vi "Handle SUBSCRIBED.vi"(0 "reference":refnum<class "WAMP Client.lvclass">, 5 "WAMP Message":T1 {"Message Codes" items=["HELLO"=1, "WELCOME"=2, "ABORT"=3, "GOODBYE"=6, "ERROR"=8, "PUBLISH"=16, "PUBLISHED"=17, "SUBSCRIBE"=32, "SUBSCRIBED"=33, "UNSUBSCRIBE"=34, "UNSUBSCRIBED"=35, "EVENT"=36, "CALL"=48, "RESULT"=59, "REGISTER"=64, "REGISTERED"=65, "UNREGISTER"=66, "UNREGISTERED"=67, "INVOCATION"=68, "YIELD"=70]}, 9 "Subscription Requests In":T3, 11 "error in (no error)":errorcluster) -> (4 "reference out":refnum<class "WAMP Client.lvclass">, 10 "Message Loop Data (out)":T3, 15 "error out":errorcluster)   [LabVIEW 2020, in "wamplv.lvlib" / "WAMP Client.lvclass"]
uses:
  WAMP Client.lvclass
  TypeDef/Message Loop Shift Reg Data.ctl
  TypeDef/REGISTER Request Data.ctl
  TypeDef/Success or error.ctl
  TypeDef/Combined error.ctl
  TypeDef/WAMP Error Payload.ctl
  TypeDef/INVOCATION payload.ctl
  TypeDef/Publish Requests Map.ctl
  TypeDef/PUBLISH Request Data.ctl
  TypeDef/PUBLISH Result.ctl
  TypeDef/Endpoint Data.ctl
  TypeDef/CALL Request Map.ctl
  TypeDef/CALL Request Data.ctl
  TypeDef/RESULT Payload.ctl
  TypeDef/SUBSCRIBE Requests Map.ctl
  TypeDef/SUBSCRIBE Request Data.ctl
  TypeDef/Subscribe Result.ctl
  TypeDef/Event Payload.ctl
  TypeDef/Subscriptions Map.ctl
  TypeDef/Subscription Details.ctl
  TypeDef/Unsubscribe Requests Map.ctl
  TypeDef/UNSUBSCRIBE Request Data.ctl
  TypeDef/UNSUBSCRIBE Result.ctl
  TypeDef/Unregister requests map.ctl
  TypeDef/Unregister request.ctl
  TypeDef/WAMP Received Message.ctl
  TypeDef/WAMP Message Codes.ctl
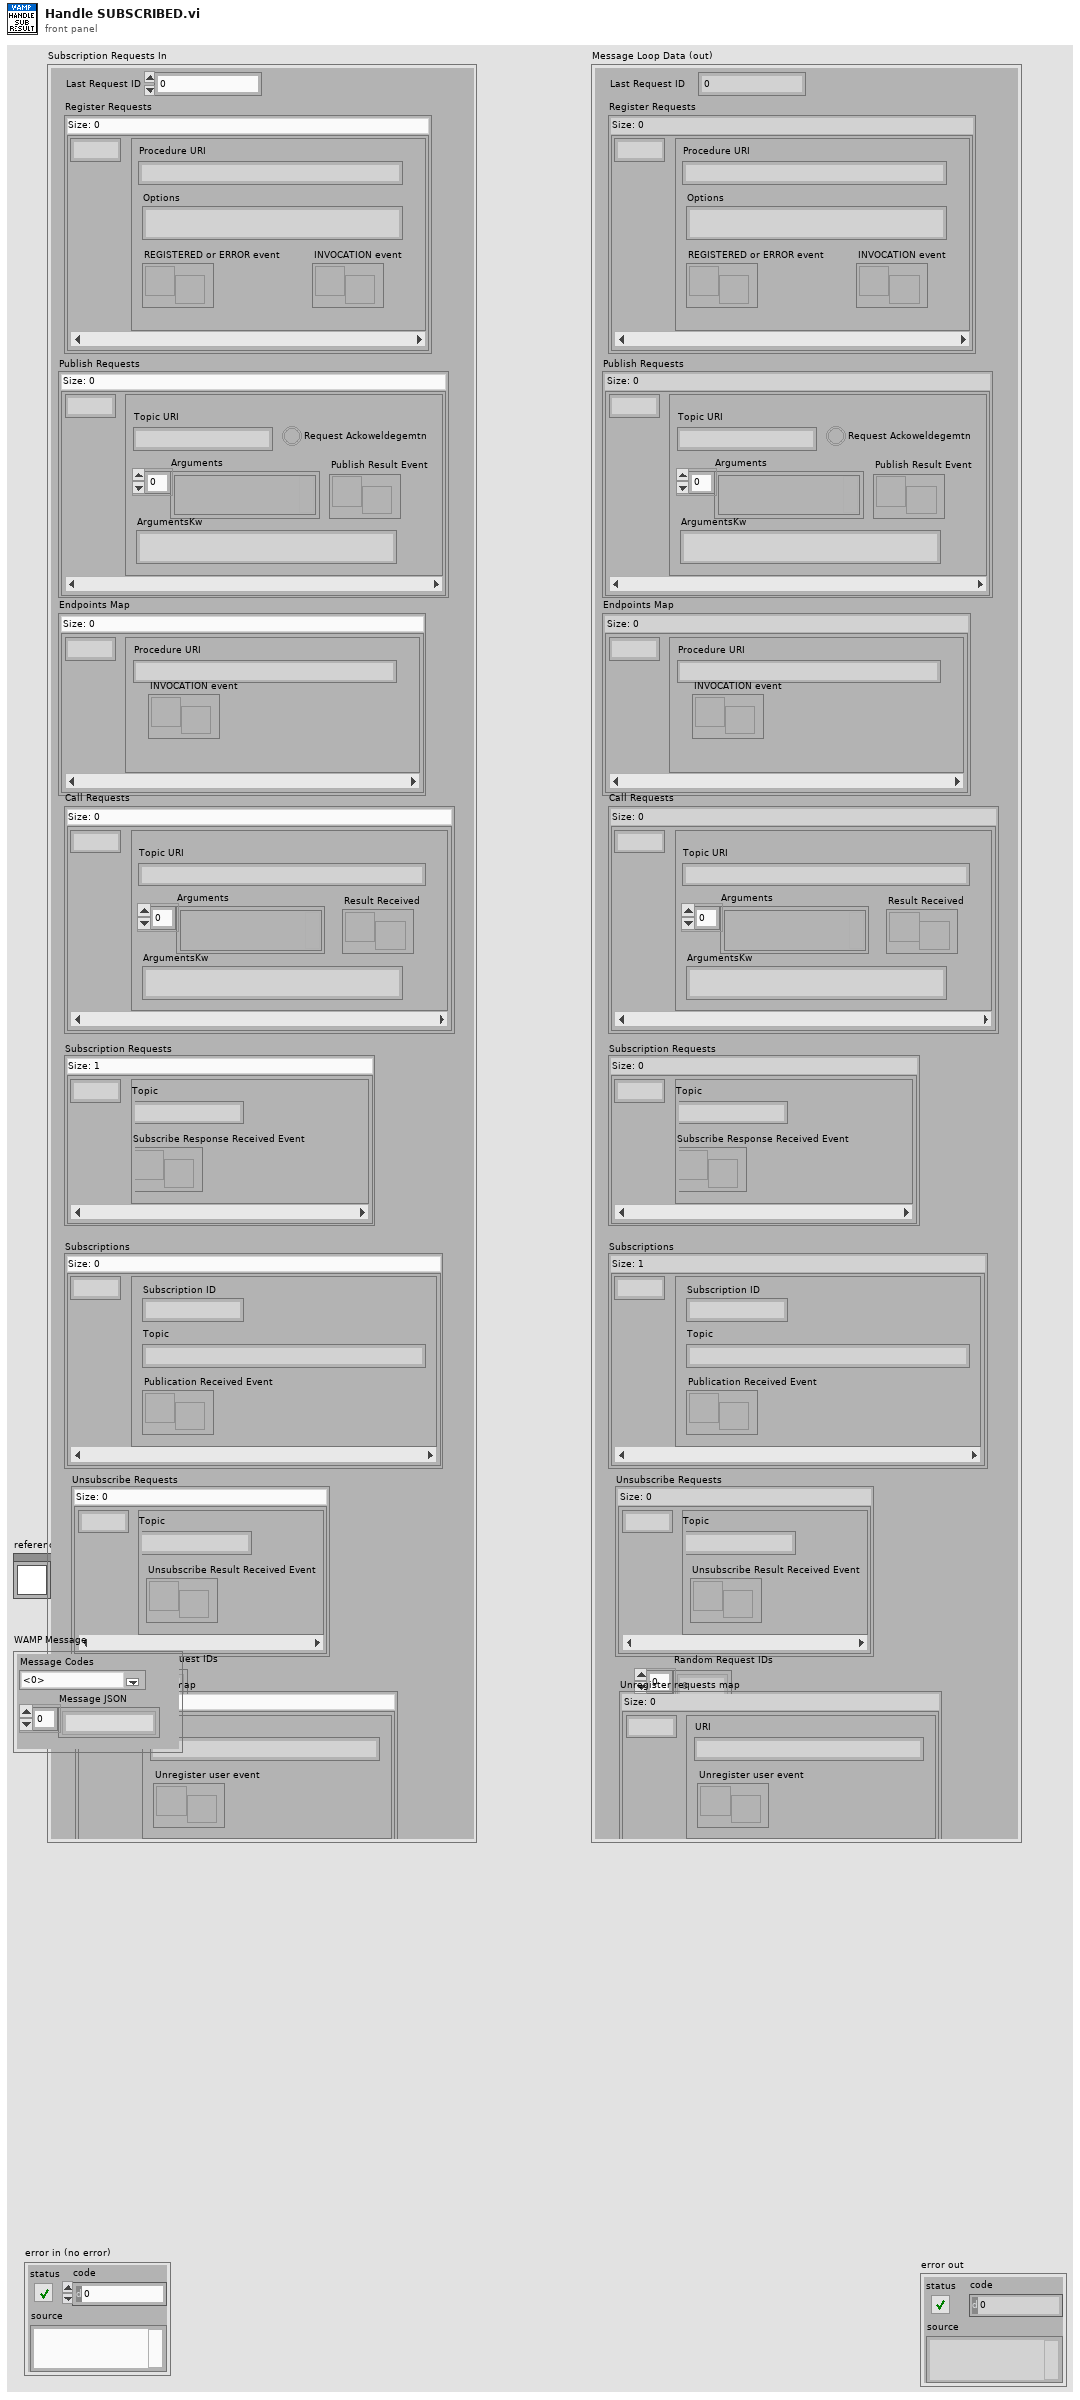
[diagram p1: front panel]
types:
  T1 = typedef "wamplv.lvlib/WAMP Client.lvclass/WAMP Received Message.ctl" = cluster{"Message JSON":string[], "Message Codes":T2}
  T2 = typedef "wamplv.lvlib/WAMP Client.lvclass/WAMP Message Codes.ctl" = u16
  T3 = typedef "wamplv.lvlib/WAMP Client.lvclass/Message Loop Shift Reg Data.ctl" = cluster{"Last Request ID":u64, "Register Requests":map{u64, T4}, "Publish Requests":T5, "Endpoints Map":map{u64, T7}, "Call Requests":T8, "Subscription Requests":T10, "Subscriptions":T12, "Unsubscribe Requests":T14, "Random Request IDs":u64[], "Unregister requests map":T16}
  T4 = typedef "wamplv.lvlib/WAMP Client.lvclass/REGISTER Request Data.ctl" = cluster{"Procedure URI":string, "Options":string, "REGISTERED or ERROR event":refnum<user-event>, "INVOCATION event":refnum<user-event>}
  T5 = typedef "wamplv.lvlib/WAMP Client.lvclass/Publish Requests Map.ctl" = map{u64, T6}
  T6 = typedef "wamplv.lvlib/WAMP Client.lvclass/PUBLISH Request Data.ctl" = cluster{"Topic URI":string, "Arguments":variant[], "ArgumentsKw":string, "Publish Result Event":refnum<user-event>, "Request Ackoweldegemtn":bool}
  T7 = typedef "wamplv.lvlib/WAMP Client.lvclass/Endpoint Data.ctl" = cluster{"Procedure URI":string, "INVOCATION event":refnum<user-event>}
  T8 = typedef "wamplv.lvlib/WAMP Client.lvclass/CALL Request Map.ctl" = map{u64, T9}
  T9 = typedef "wamplv.lvlib/WAMP Client.lvclass/CALL Request Data.ctl" = cluster{"Topic URI":string, "Arguments":variant[], "ArgumentsKw":string, "Result Received":refnum<user-event>}
  T10 = typedef "wamplv.lvlib/WAMP Client.lvclass/SUBSCRIBE Requests Map.ctl" = map{u64, T11}
  T11 = typedef "wamplv.lvlib/WAMP Client.lvclass/SUBSCRIBE Request Data.ctl" = cluster{"Topic":string, "Subscribe Response Received Event":refnum<user-event>}
  T12 = typedef "wamplv.lvlib/WAMP Client.lvclass/Subscriptions Map.ctl" = map{u64, T13}
  T13 = typedef "wamplv.lvlib/WAMP Client.lvclass/Subscription Details.ctl" = cluster{"Subscription ID":u64, "Topic":string, "Publication Received Event":refnum<user-event>}
  T14 = typedef "wamplv.lvlib/WAMP Client.lvclass/Unsubscribe Requests Map.ctl" = map{u64, T15}
  T15 = typedef "wamplv.lvlib/WAMP Client.lvclass/UNSUBSCRIBE Request Data.ctl" = cluster{"Topic":string, "Unsubscribe Result Received Event":refnum<user-event>}
  T16 = typedef "wamplv.lvlib/WAMP Client.lvclass/Unregister requests map.ctl" = map{u64, T17}
  T17 = typedef "wamplv.lvlib/WAMP Client.lvclass/Unregister request.ctl" = cluster{"URI":string, "Unregister user event":refnum<user-event>}
  T18 = typedef "wamplv.lvlib/WAMP Client.lvclass/Subscribe Result.ctl" = cluster{"Success?":bool, "Publication Received Event":refnum<user-event>, "Combined Error":T19}
  T19 = typedef "wamplv.lvlib/WAMP Client.lvclass/Combined error.ctl" = cluster{"Error?":bool, "WAMP Error":T20, "Error":errorcluster}
  T20 = typedef "wamplv.lvlib/WAMP Client.lvclass/WAMP Error Payload.ctl" = cluster{"Details":string, "ArgumentKw Payload":string, "Wamp error?":bool, "Error URI":string, "Arguments Payload":string[]}
  T21 = typedef "wamplv.lvlib/WAMP Client.lvclass/Event Payload.ctl" = cluster{"Arguments Payload":string[], "ArgumentKw Payload":string, "Topic":string}
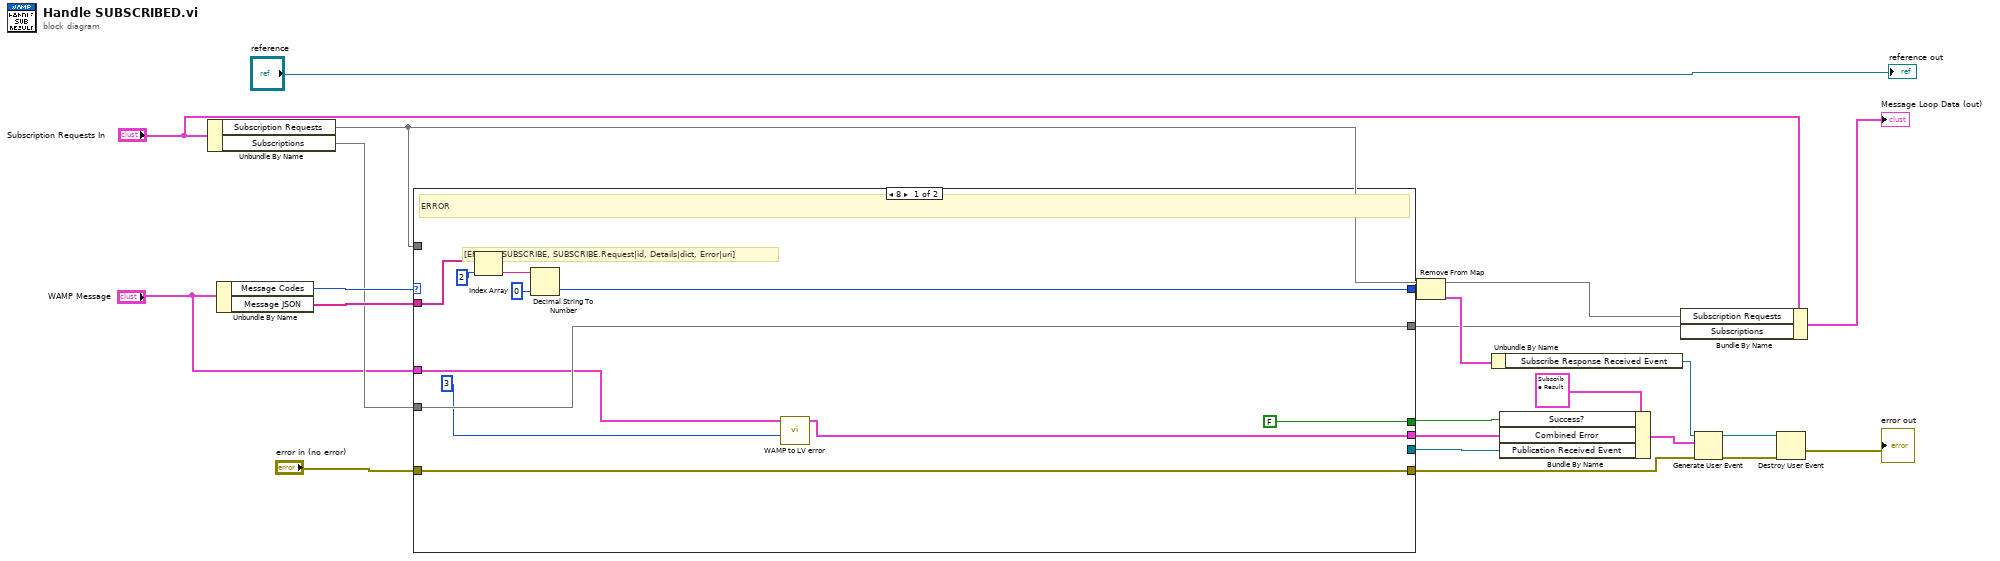
[diagram p0: block diagram]
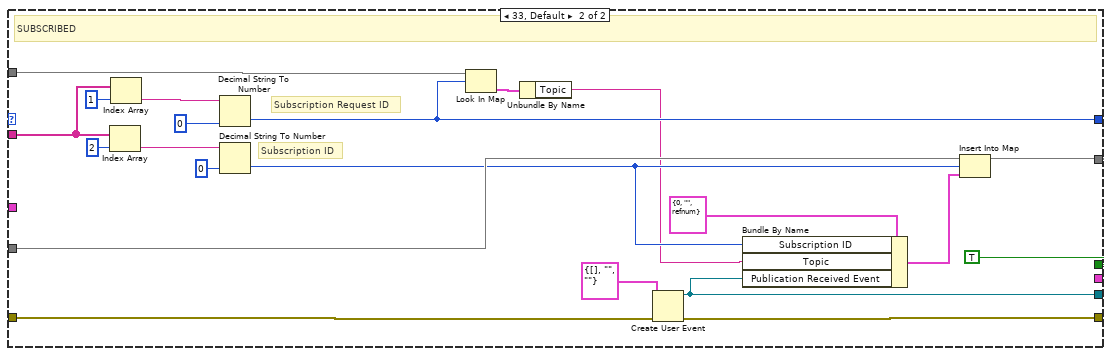
[diagram p2: hidden frame]
diagram:
  n1 = Unbundle By Name("Subscription Requests In") -> ("Subscription Requests"=w9:T10, "Subscriptions"=w8:T12)
  n2 = Unbundle By Name("WAMP Message") -> ("Message Codes"=w18:T2, "Message JSON"=w17:string[])
  n3 = case shown="8" w18 {
    tunnel: w17 -> [w32 w52]
    tunnel: [w30 w42] -> w16
    tunnel: "error in (no error)" -> [w24 w36]
    tunnel: [w24 w35] -> w1
    tunnel: [FALSE ("Success?") TRUE ("Success?")] -> w21
    tunnel: w8 -> [w29 w47]
    tunnel: w9 -> [_ w43]
    tunnel: [w29 w38] -> w4
    tunnel: [_ w37] -> w10
    tunnel: [w25 _] -> w3
    tunnel: "WAMP Message" -> [w26 _]
    frame 8 {
      # "[ERROR, SUBSCRIBE, SUBSCRIBE.Request|id, Details|dict, Error|uri]"
      # "ERROR"
      n4 = Index Array(array=w32, index=2) -> (element=w33:string)
      n5 = Decimal String To Number(string=w33, default (0L)=u64 0 ("default (0 I32)")) -> (number=w30:u64)  [unwired: 1 in, 1 out]
      n6 = call "WAMP to LV error.vi"("Details Index"=u32 3, "WAMP Message"=w26) -> ("Combined Error"=w25:T19)  [unwired: 7 in, 2 out]
    }
    frame 33, Default {
      # "Subscription Request ID"
      # "Subscription ID"
      # "SUBSCRIBED"
      n7 = Index Array(array=w52, index=2) -> (element=w54:string)
      n8 = Index Array(array=w52, index=1) -> (element=w50:string)
      n9 = Decimal String To Number(string=w50, default (0L)=u64 0) -> (number=w42:u64)  [unwired: 1 in, 1 out]
      n10 = Decimal String To Number(string=w54, default (0L)=u64 0) -> (number=w45:u64)  [unwired: 1 in, 1 out]
      n11 = Look In Map(map=w43, key=w42) -> (value=w41:T11)  [unwired: 1 in, 1 out]
      n12 = Unbundle By Name(w41) -> ("Topic"=w40:string)
      n13 = Create User Event(user event datatype=T21 {"Arguments Payload"=[], "ArgumentKw Payload"="", "Topic"=""} ("Cluster"), error in=w36) -> (user event=w37:refnum<user-event>, error out=w35:errorcluster)
      n14 = Bundle By Name(cluster=T13 {"Subscription ID"=0, "Topic"="", "Publication Received Event"=refnum} ("Cluster"), "Subscription ID"=w45, "Topic"=w40, "Publication Received Event"=w37) -> (w44:T13)
      n15 = Insert Into Map(map in=w47, key=w45, value=w44) -> (map out=w38:T12)  [unwired: 2 out]
    }
  }
  n16 = Remove From Map(10:w16, 11:w9) -> (1:w15:T11, 3:w7:T10)  [unwired: 1 out]
  n17 = Unbundle By Name(w15) -> ("Subscribe Response Received Event"=w14:refnum<user-event>)
  n18 = Bundle By Name(cluster=T18 {"Success?"=FALSE, "Publication Received Event"=refnum, "Combined Error"={"Error?"=FALSE, "WAMP Error"={"Details"="", "ArgumentKw Payload"="{}", "Wamp error?"=FALSE, "Error URI"="", "Arguments Payload"=[]}, "Error"={"status"=FALSE, "code"=0, "source"=""}}} ("event data"), "Success?"=w21, "Combined Error"=w3, "Publication Received Event"=w10) -> (w20:T18)
  n19 = Bundle By Name(cluster="Subscription Requests In", "Subscription Requests"=w7, "Subscriptions"=w4) -> (→"Message Loop Data (out)":T3)
  n20 = Generate User Event(user event=w14, event data cluster=w20, error in=w1) -> (user event out=w11:refnum<user-event>, error out=w13:errorcluster)  [unwired: 1 in]
  n21 = Destroy User Event(user event=w11, error in=w13) -> (error out=→"error out":errorcluster)
  "reference out" <- "reference"
